vi "write_custom_timestamp.vi"(8 "error in (no error)":errorcluster, 10 "timestamp (ns)":u64, 11 "Refnum in":T1) -> (0 "error out":errorcluster, 3 "Refnum out":T1)   [LabVIEW 2020, in "MagSpecStitcher.lvclass"]
uses:
  MagSpecStitcher.lvclass
  <vilib>/vision/Image Controls.llb/IMAQ Image.ctl
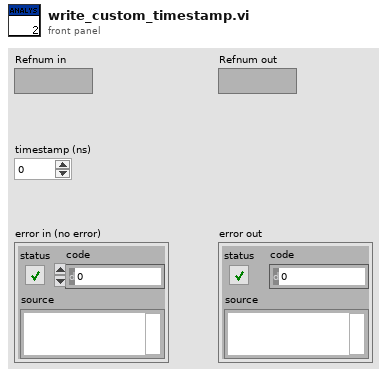
[diagram p1: front panel]
types:
  T1 = typedef "IMAQ Image.ctl" = refnum<image>
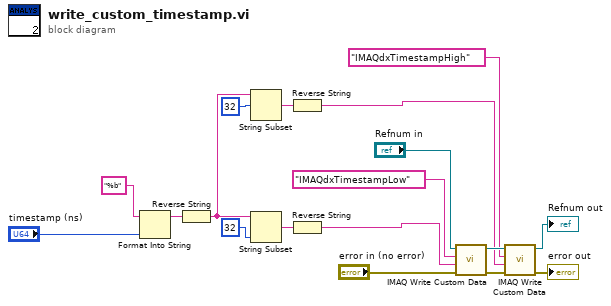
[diagram p0: block diagram]
diagram:
  n1 = Format Into String(format string="%b", "timestamp (ns)") -> (resulting string=w4:string)  [unwired: 2 in, 1 out]
  n2 = Reverse String(1:w4) -> (0:w6:string)
  n3 = String Subset(string=w6, offset (0)=32) -> (substring=w9:string)  [unwired: 1 in]
  n4 = String Subset(string=w6, length (rest)=32 ("length (rest)")) -> (substring=w8:string)  [unwired: 1 in]
  n5 = Reverse String(1:w9) -> (0:w1:string)
  n6 = Reverse String(1:w8) -> (0:w2:string)
  n7 = call "IMAQ Write Custom Data"("error in (no error)"="error in (no error)", "Custom Data In"=w2, "Key"="IMAQdxTimestampLow", "Image"="Refnum in") -> ("error out"=w15:errorcluster, "Image Out"=w14:T1)  [unwired: 6 in]
  n8 = call "IMAQ Write Custom Data"("error in (no error)"=w15, "Custom Data In"=w1, "Key"="IMAQdxTimestampHigh", "Image"=w14) -> ("error out"=→"error out":errorcluster, "Image Out"=→"Refnum out":T1)  [unwired: 6 in]
